vi "Draw ANN configuration.vi"(0 "Array":i16[](array[numeric])) -> (1 "Xmax":i8, 2 "Ymax":i16, 3 "Map of the neural network (node configuration)":cluster{dbl[], dbl[]}[](graph))   [LabVIEW 2010]
panel:
  out "No of neurons":i8
  out "Hidden 6":i8 min=0 max=20 step=1
  out "Hidden 5":i8 min=0 max=20 step=1
  out "Hidden 4":i8 min=0 max=20 step=1
  out "Outputs":i8=1 min=1 max=20 step=1
  out "Hidden 3":i8 min=0 max=20 step=1
  out "Hidden 2":i8 min=0 max=20 step=1
  out "Hidden 1":i8=1 min=1 max=20 step=1
  out "Inputs":i8=1 min=1 max=20 step=1
  # "Hidden layers"
  # "Outputs"
  # "Inputs"
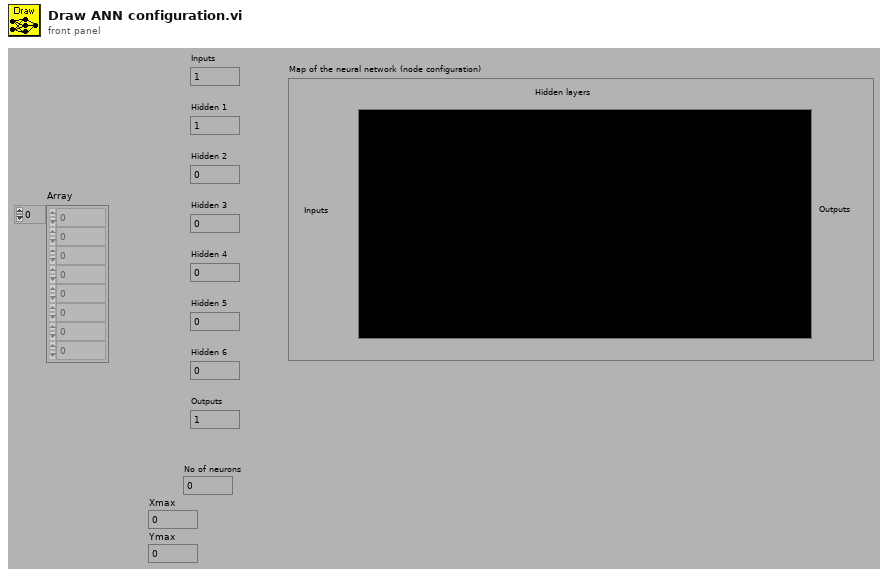
[diagram p1: front panel]
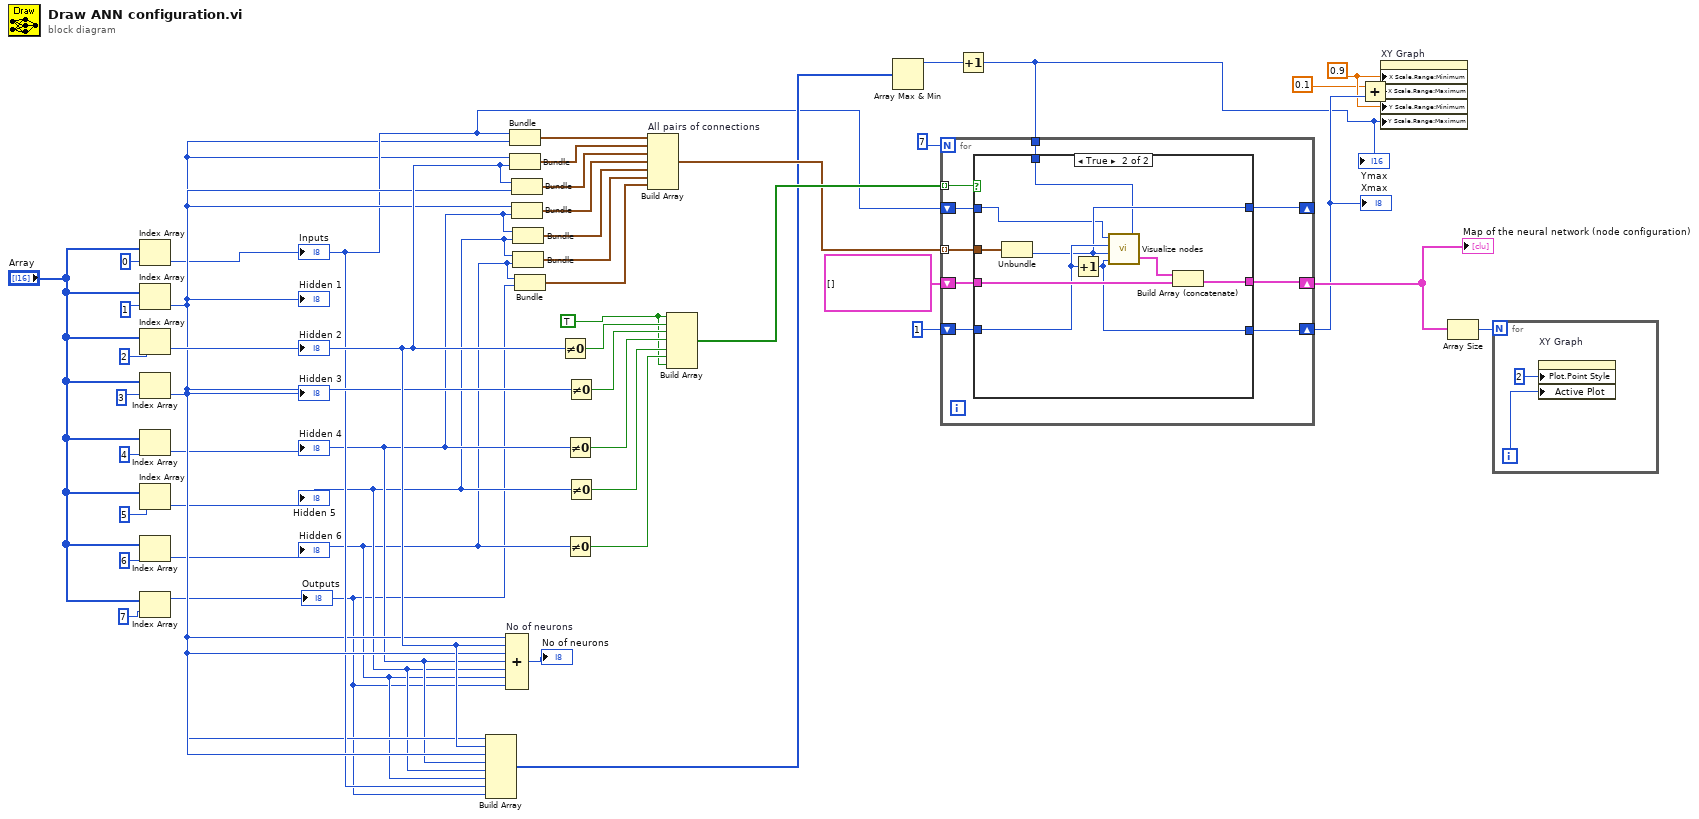
[diagram p0: block diagram]
diagram:
  w23 = 0.9
  w39 = TRUE
  n1 = Index Array(array="Array", index=0 ("Index")) -> (element=w13:i16)
  "Inputs" <- w13
  n2 = Index Array(array="Array", index=1 ("Index")) -> (element=w12:i16)
  "Hidden 1" <- w12
  n3 = Index Array(array="Array", index=2 ("Index")) -> (element=w19:i16)
  "Hidden 2" <- w19
  n4 = Index Array(array="Array", index=3 ("Index")) -> (element=w18:i16)
  "Hidden 3" <- w18
  n5 = Index Array(array="Array", index=4 ("Index")) -> (element=w4:i16)
  "Hidden 4" <- w4
  n6 = Index Array(array="Array", index=5 ("Index")) -> (element=w3:i16)
  "Hidden 5" <- w3
  n7 = Index Array(array="Array", index=6 ("Index")) -> (element=w2:i16)
  "Hidden 6" <- w2
  n8 = Index Array(array="Array", index=7 ("Index")) -> (element=w1:i16)
  "Outputs" <- w1
  n9 = Build Array(w12, w19, w18, w4, w3, w2, w13, w1) -> (w16:i16[])
  n10 = Compound Arithmetic op=ADD "No of neurons"(w12, w19, w18, w4, w3, w2, w1) -> (→"No of neurons":i16)
  n11 = Bundle("Numeric"=w13, "Numeric"=w12) -> (w37:cluster{"Numeric":i16, "Numeric":i16})  [unwired: 1 in]
  n12 = Bundle("Numeric"=w12, "Numeric"=w19) -> (w36:cluster{"Numeric":i16, "Numeric":i16})  [unwired: 1 in]
  n13 = Bundle("Numeric"=w19, "Numeric"=w18) -> (w35:cluster{"Numeric":i16, "Numeric":i16})  [unwired: 1 in]
  n14 = Bundle("Numeric"=w18, "Numeric"=w4) -> (w34:cluster{"Numeric":i16, "Numeric":i16})  [unwired: 1 in]
  n15 = Bundle("Numeric"=w4, "Numeric"=w3) -> (w33:cluster{"Numeric":i16, "Numeric":i16})  [unwired: 1 in]
  n16 = Bundle("Numeric"=w3, "Numeric"=w2) -> (w32:cluster{"Numeric":i16, "Numeric":i16})  [unwired: 1 in]
  n17 = Bundle("Numeric"=w2, "Numeric"=w1) -> (w31:cluster{"Numeric":i16, "Numeric":i16})  [unwired: 1 in]
  n18 = Not Equal To 0?(x=w19) -> (x != 0?=w44:bool)
  n19 = Not Equal To 0?(x=w4) -> (x != 0?=w42:bool)
  n20 = Not Equal To 0?(x=w2) -> (x != 0?=w40:bool)
  n21 = Not Equal To 0?(x=w18) -> (x != 0?=w43:bool)
  n22 = Not Equal To 0?(x=w3) -> (x != 0?=w41:bool)
  n23 = Build Array "All pairs of connections"(w37, w36, w35, w34, w33, w32, w31) -> (w17:cluster{"Numeric":i16, "Numeric":i16}[])
  n24 = Build Array(w39, w44, w43, w42, w41, w40, w39) -> (w38:bool[])
  n25 = Array Max & Min(array=w16) -> (max value=w24:i16)  [unwired: 3 out]
  n26 = Increment(x=w24) -> (x+1=w21:i16)
  "Ymax" <- w21
  n27 = for {
    N: 7 -> [_]
    tunnel: w38 -> [w54] mode=indexing
    tunnel: w17 -> [w53] mode=indexing
    shift-right: [w52] -> w28
    shift-left: cluster{dbl[], dbl[]}[] [] -> [w51]
    shift-right: [w49] -> w26
    shift-left: i8 1 -> [w50]
    shift-right: [w48] -> _
    shift-left: w13 -> [w47]
    tunnel: w21 -> [w46]
    n28 = case shown="True" w54 {
      tunnel: w53 -> [_ w66]
      tunnel: [w57 w64] -> w52
      tunnel: w51 -> [w57 w63]
      tunnel: w50 -> [w56 w62]
      tunnel: [w56 w61] -> w49
      tunnel: [w55 w60] -> w48
      tunnel: w47 -> [w55 w59]
      tunnel: w46 -> [_ w58]
      frame False {
      }
      frame True {
        n29 = Unbundle(w66) -> ("Numeric"=w60:i16)  [unwired: 1 out]
        n30 = Increment(x=w62) -> (x+1=w61:i8)
        n31 = call "Visualize nodes.vi"("Max number (for centering)"=w58, "X 2"=w61, "Nodes 2"=w60, "X 1"=w62, "Nodes 1"=w59) -> ("XY Graph"=w65:cluster{dbl[], dbl[]}[])
        n32 = Build Array (concatenate)(w65, w63) -> (w64:cluster{dbl[], dbl[]}[])
      }
    }
  }
  "Map of the neural network (node configuration)" <- w28
  "Xmax" <- w26
  n33 = Add(x=0.1, y=w26) -> (x+y=w25:dbl)
  n34 = property on="XY Graph" class="XYGraph (strict)"("X Scale.Range:Minimum"=w23, "X Scale.Range:Maximum"=w25, "Y Scale.Range:Minimum"=w23, "Y Scale.Range:Maximum"=w21) -> ()  [unwired: 2 in, 2 out]
  n35 = Array Size(array=w28) -> (size(s)=w27:i32)
  n36 = for {
    N: w27 -> [_]
    i -> [w67]
    n37 = property on="XY Graph" class="XYGraph (strict)"("Plot.Point Style"=u8 2 ("Write Attribute"), "Active Plot"=w67) -> ()  [unwired: 2 in, 2 out]
  }
